vi "DAQinput.vi"() -> ()   [LabVIEW 2018]
panel:
  in  "停止":bool
  out "波形图":dynamicdata(graph)
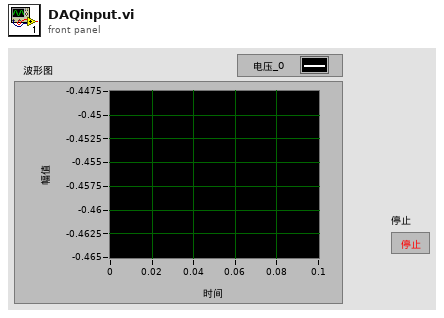
[diagram p1: front panel]
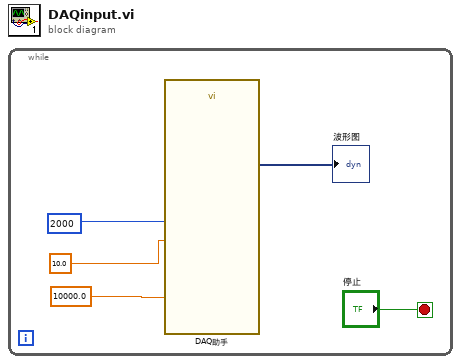
[diagram p0: block diagram]
diagram:
  n1 = while {
    stop <- "停止" stop-if-true
    n2 = call "DAQ助手"("速率"=10000.0, "采样数"=2000, "timeout (s)"=10.0) -> ("data"=→"波形图":dynamicdata)  [unwired: 14 in, 2 out]
  }
